vi "Read Action.vi"(11 "ActionStack in":refnum<class "Stack.lvclass">) -> (2 "Action":string, 3 "ActionStack out":refnum<class "Stack.lvclass">)   [LabVIEW 2025]
uses:
  Stack.lvclass/Stack.ctl
  Stack.lvclass
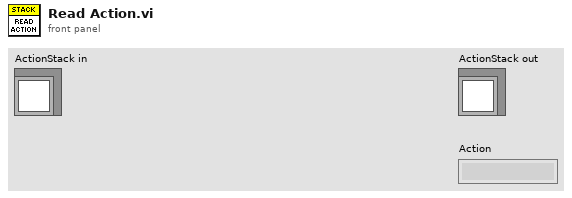
[diagram p1: front panel]
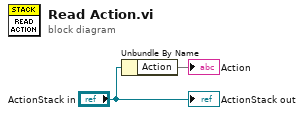
[diagram p0: block diagram]
diagram:
  n1 = Unbundle By Name("ActionStack in") -> ("Action"=→"Action")
  "ActionStack out" <- "ActionStack in"
